vi "Stop Core.vi"(10 "final error code":i32, 11 "Controller in":refnum<class "Controller.lvclass">) -> (3 "Controller out":refnum<class "Controller.lvclass">)   [LabVIEW 2026, in "Controller Actor.lvlib" / "Controller.lvclass"]
uses:
  Controller.lvclass
  Controller.lvclass/Controller.ctl
  <vilib>/ActorFramework/Message Enqueuer/Message Enqueuer.lvclass/Message Enqueuer.ctl
  <vilib>/ActorFramework/Message Enqueuer/Enqueue.vi
  <vilib>/ActorFramework/Stop Msg/Stop Msg.lvclass
  User Interface/Messages/Disable UI Msg/Disable UI Msg.lvclass
  <vilib>/ActorFramework/Message Priority Queue/Priority Enqueue.vi
  <vilib>/ActorFramework/Message Enqueuer/Message Enqueuer.lvclass
  <vilib>/ActorFramework/Actor/Actor.lvclass
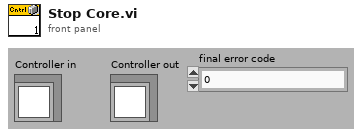
[diagram p1: front panel]
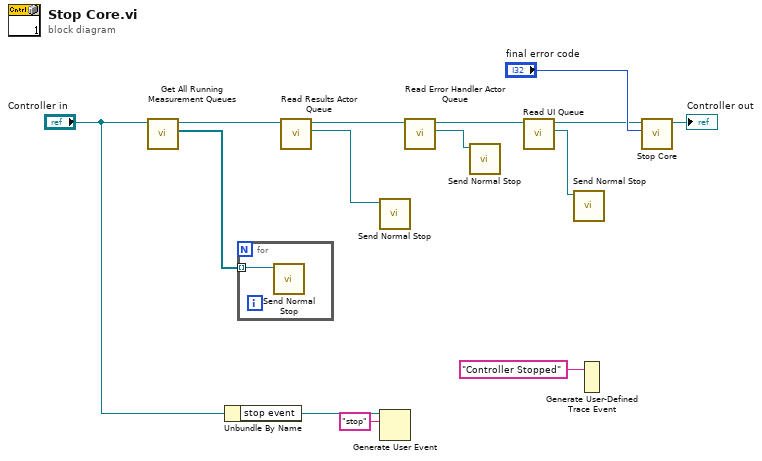
[diagram p0: block diagram]
diagram:
  n1 = call "Get All Running Measurement Queues.vi"("Controller in"="Controller in") -> ("Array of Measurement Queues"=w13:refnum<class "Message Enqueuer.lvclass">[], "Controller out"=w12:refnum<class "Controller.lvclass">)  [unwired: 8 in, 1 out]
  n2 = Unbundle By Name("Controller in") -> ("stop event"=w2:refnum<user-event>)
  n3 = for {
    tunnel: w13 -> [w15] mode=indexing
    n4 = call <vilib>:"Send Normal Stop.vi"("Message Enqueuer"=w15) -> ()  [unwired: 10 in, 1 out]
  }
  n5 = call "Read Results Actor Queue.vi"("Controller in"=w12) -> ("Message Enqueuer"=w11:refnum<class "Message Enqueuer.lvclass">, "Controller out"=w9:refnum<class "Controller.lvclass">)  [unwired: 8 in, 1 out]
  n6 = call <vilib>:"Send Normal Stop.vi"("Message Enqueuer"=w11) -> ()  [unwired: 10 in, 1 out]
  n7 = Generate User Event(user event=w2, event data cluster="stop" ("event data")) -> ()  [unwired: 2 in, 2 out]
  n8 = call "Read Error Handler Actor Queue.vi"("Controller in"=w9) -> ("Actor Framework.lvlib:Message Enqueuer"=w8:refnum<class "Message Enqueuer.lvclass">, "Controller out"=w6:refnum<class "Controller.lvclass">)  [unwired: 8 in, 1 out]
  n9 = call <vilib>:"Send Normal Stop.vi"("Message Enqueuer"=w8) -> ()  [unwired: 10 in, 1 out]
  n10 = call "Read UI Queue.vi"("UI Controller in"=w6) -> ("UI Queue"=w4:refnum<class "Message Enqueuer.lvclass">, "UI Controller out"=w5:refnum<class "Controller.lvclass">)  [unwired: 8 in, 1 out]
  n11 = call <vilib>:"Send Normal Stop.vi"("Message Enqueuer"=w4) -> ()  [unwired: 10 in, 1 out]
  n12 = Generate User-Defined Trace Event(2:"Controller Stopped" ("trace string")) -> ()  [unwired: 1 in]
  n13 = call-parent "Stop Core.vi"("final error code"="final error code", "Actor in"=w5) -> ("Actor out"=→"Controller out":refnum<class "Controller.lvclass">)  [unwired: 9 in]
